vi "serial_mvmnt_init.vi"(0 "error in":errorcluster) -> (1 "System no.":i32=1, 2 "error out":errorcluster, 3 "Conn. Axes":string[](array[string]))   [LabVIEW 2016]
panel:
  out "Running":bool caption="Configuration_Setup.vi is running"
  out "Identification":string
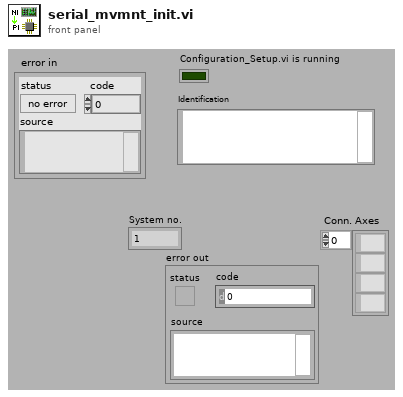
[diagram p1: front panel]
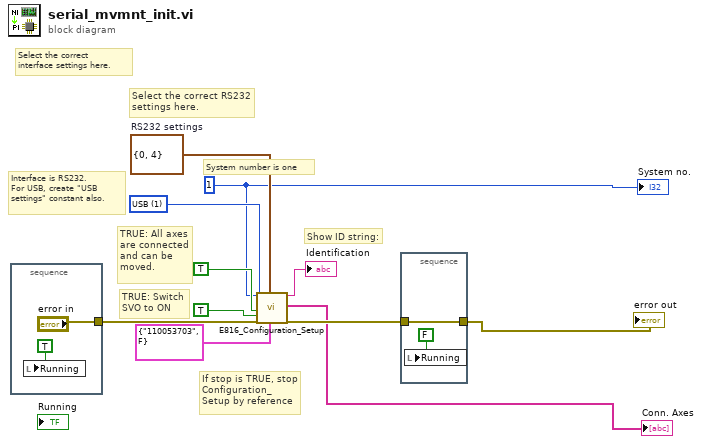
[diagram p0: block diagram]
diagram:
  w3 = u16 1 items=["RS232", "USB"] ("Interface")
  w6 = cluster{"Portnumber":i32, "Baudrate":u16} {"Portnumber"=0, "Baudrate"=4}  # RS232 settings
  w2 = 1 ("System no.")
  # "Select the correct\ninterface settings here."
  # "Interface is RS232.\nFor USB, create \"USB\nsettings\" constant also."
  # "TRUE: All axes\nare connected\nand can be\nmoved."
  # "TRUE: Switch\nSVO to ON"
  # "If stop is TRUE, stop\nConfiguration_\nSetup by reference"
  # "Select the correct RS232\nsettings here."
  # "Show ID string:"
  # "System number is one"
  n1 = stacked-sequence {
    tunnel: ["error in"] -> w9
    frame #0 {
      n2 = local write "Running"(TRUE ("Running")) -> ()
    }
  }
  n3 = call "E816_Configuration_Setup.vi"("System no."=w2, "Interface"=w3, "All axes?"=TRUE, "Change servo \nstatus to ON?"=TRUE ("Use dialog to define\nconnected stages?"), "error in"=w9, "RS232 settings"=w6, "USB settings"=cluster{"S/N":string, "USB Search?":bool} {"S/N"="110053703", "USB Search?"=FALSE}) -> ("Identification"=→"Identification":string, "Conn. Axes"=→"Conn. Axes":string[], "error out"=w10:errorcluster)  [unwired: 4 in, 6 out]
  n4 = stacked-sequence {
    tunnel: w10 -> [w15]
    tunnel: [w15] -> w8
    frame #0 {
      n5 = local write "Running"(FALSE ("Running")) -> ()
    }
  }
  "error out" <- w8
  "System no." <- w2
